vi "InitShooter.vi"   [LabVIEW 2020]
doc: "This VI initializes devices related directly to the shooter subsystem."
uses:
  <vilib>/Rock Robotics/WPI/ThirdParty/Phoenix-LabVIEW/Motor Controller/Controls/CTRE_Phoenix_MotorControl_NeutralMode.ctl
  <vilib>/Rock Robotics/WPI/ThirdParty/Phoenix-LabVIEW/Motor Controller/Controls/CTRE_Phoenix_MotorControl_TalonFXInvertType.ctl
  <vilib>/Rock Robotics/WPI/ThirdParty/Phoenix-LabVIEW/Motor Controller/Controls/CTRE_Phoenix_MotorControl_SupplyCurrentLimitConfiguration.ctl
  <vilib>/Rock Robotics/WPI/ThirdParty/Phoenix-LabVIEW/Motor Controller/Controls/CTRE_Phoenix_MotorControl_FeedbackDevice_TalonFX.ctl
  <vilib>/Rock Robotics/WPI/ThirdParty/Phoenix-LabVIEW/Motor Controller/Controls/CTRE_Phoenix_MotorControl_LimitSwitchSource_Local.ctl
  <vilib>/Rock Robotics/WPI/ThirdParty/Phoenix-LabVIEW/Motor Controller/Controls/CTRE_Phoenix_MotorControl_LimitSwitchNormal.ctl
  <vilib>/Rock Robotics/WPI/ThirdParty/Phoenix-LabVIEW/Motor Controller/Controls/CTRE_Phoenix_MotorControl_StatusFrameEnhanced.ctl
  refnumbers.vi
  robotconstants.vi
types:
  T1 = typedef "CTRE_Phoenix_MotorControl_StatusFrameEnhanced.ctl" = u16
  T2 = typedef "CTRE_Phoenix_MotorControl_LimitSwitchNormal.ctl" = enum16{"Normally Open", "Normally Closed", "Disabled"}
  T3 = typedef "CTRE_Phoenix_MotorControl_LimitSwitchSource_Local.ctl" = enum16{"Feedback Connector", "Remote Talon SRX", "Remote CANifier", "Deactivated"}
  T4 = typedef "CTRE_Phoenix_MotorControl_FeedbackDevice_TalonFX.ctl" = i8
  T5 = typedef "CTRE_Phoenix_MotorControl_SupplyCurrentLimitConfiguration.ctl" = cluster{"Enable?":bool, "Current Limit":dbl, "Threshold Current":dbl, "Threshold Time":dbl}
  T6 = typedef "CTRE_Phoenix_MotorControl_NeutralMode.ctl" = enum8{"EEPROMSetting", "Override to Coast", "Override to Brake"}
  T7 = typedef "CTRE_Phoenix_MotorControl_TalonFXInvertType.ctl" = enum16{"Counter-Clockwise", "Clockwise"}
  T8 = typedef "WPI_MotorControlDeviceRef.ctl" = cluster{"DeviceStatus":errorcluster, "Type":T9, "PWM":cluster{"PWM Channel":T10, "DeadBand":T11}, "CAN":cluster{"Device Number":u8, "SetOutput VI Ref":variant, "GetOutput VI Ref":variant, "Enable VI Ref":variant, "Disable VI Ref":variant, "Data":variant}, "Invert":bool, "DIO PWM":cluster{"PWM \"Enable\" Channel":T10, "DIOChannel":T12, "PWM Rate":dbl}}
  T9 = typedef "WPI_MotorControlType.ctl" = enum16{"PWM", "CAN", "DIO PWM"}
  T10 = typedef "FPGA_DIOPWMChannel.ctl" = enum8{"PWM 0", "PWM 1", "PWM 2", "PWM 3", "PWM 4", "PWM 5", "PWM 6", "PWM 7", "PWM 8", "PWM 9", "PWM MXP 0", "PWM MXP 1", "PWM MXP 2", "PWM MXP 3", "PWM MXP 4", "PWM MXP 5", "PWM MXP 6", "PWM MXP 7", "PWM MXP 8", "PWM MXP 9", "Invalid"}
  T11 = typedef "WPI_PWMDeadband.ctl" = cluster{"Name":string, "maxPositivePwm":i32, "minPositivePwm":i32, "centerPwm":i32, "maxNegativePwm":i32, "minNegativePwm":i32, "angularRange":u16}
  T12 = typedef "FPGA_DIOChannel.ctl" = enum8{"DIO 0", "DIO 1", "DIO 2", "DIO 3", "DIO 4", "DIO 5", "DIO 6", "DIO 7", "DIO 8", "DIO 9", "DIO MXP 0", "DIO MXP 1", "DIO MXP 2", "DIO MXP 3", "DIO MXP 4", "DIO MXP 5", "DIO MXP 6", "DIO MXP 7", "DIO MXP 8", "DIO MXP 9", "DIO MXP 10", "DIO MXP 11", "DIO MXP 12", "DIO MXP 13", "DIO MXP 14", "DIO MXP 15", "SPI Port CS1", "SPI Port CS2", "SPI Port CS3", "SPI Port MISO", "SPI Port MOSI", "Invalid"}
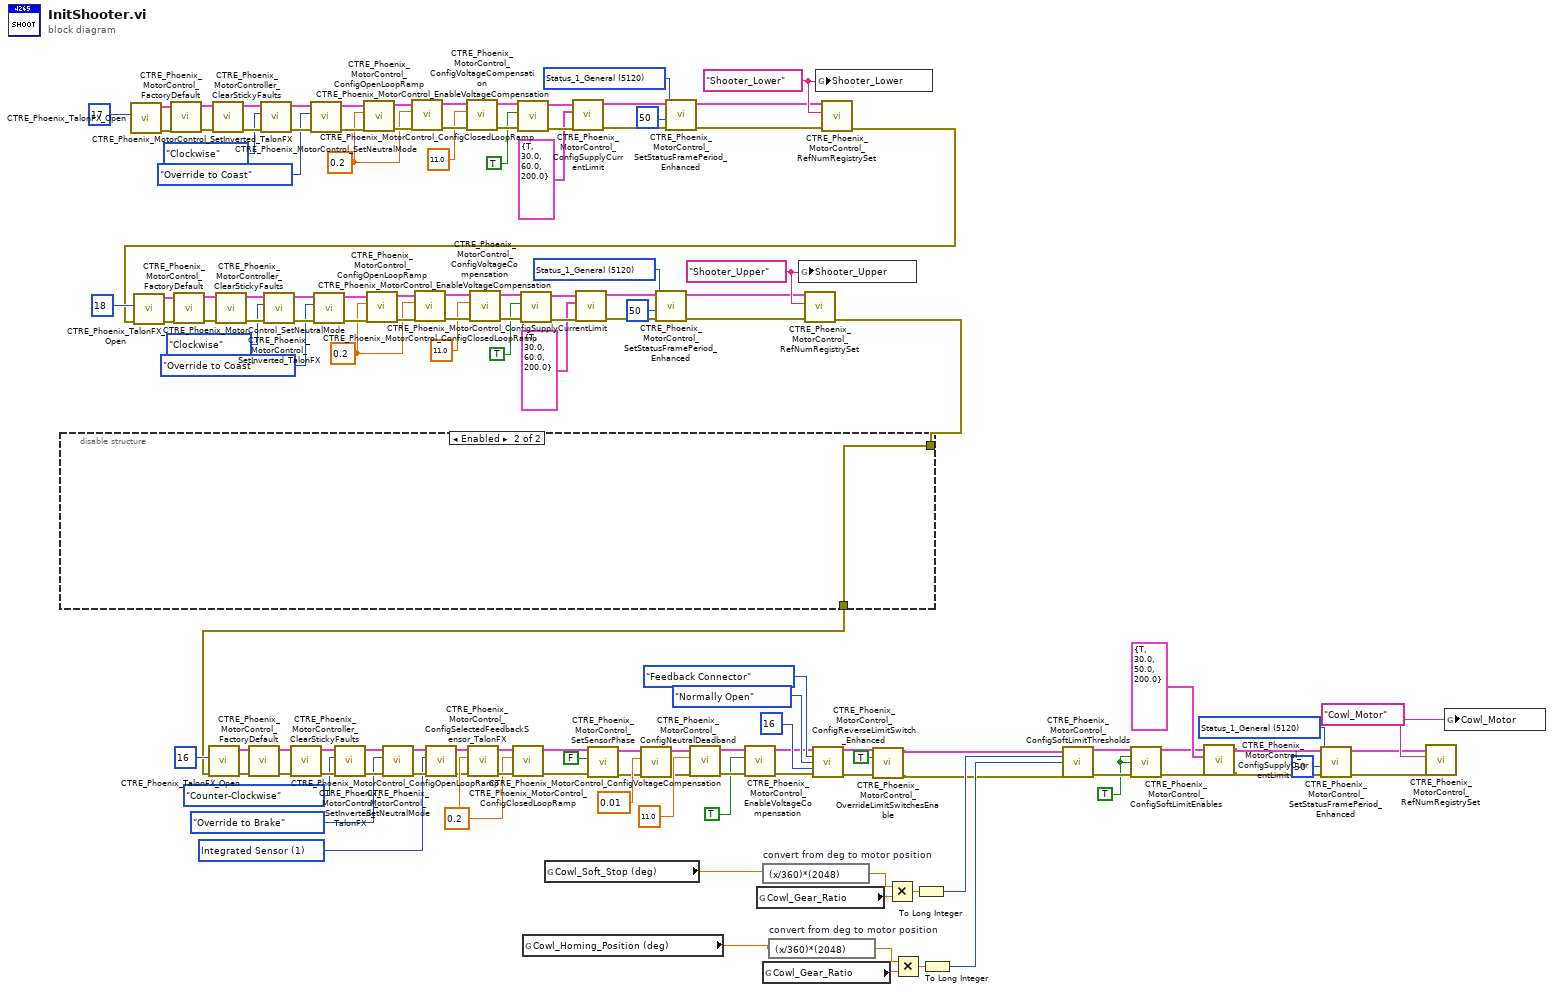
[diagram p0: block diagram]
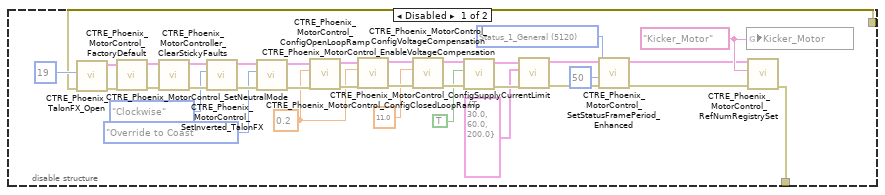
[diagram p2: hidden frame]
diagram:
  w17 = TRUE ("Forward Soft Limit Enable")
  w29 = T1 5120 items=["Status_1_General"=5120, "Status_2_Feedback0"=5184, "Status_3_Quadrature"=5248, "Status_4_AinTempVbat"=5312, "Status_6_Misc"=5440, "Status_7_CommStatus"=5504, "Status_8_PulseWidth"=5568, "Status_9_MotProfBuffer"=5632, "Status_10_MotionMagic"=5696, "Status_11_UartGadgeteer"=5760, "Status_12_Feedback1"=5824, "Status_13_Base_PIDF0"=5888, "Status_14_Turn_PIDF1"=5952, "Status_15_FirmwareApiStatus"=6016, "Status_Brushless_Current"=4672] ("Status Frame")
  w35 = T1 5120 items=["Status_1_General"=5120, "Status_2_Feedback0"=5184, "Status_3_Quadrature"=5248, "Status_4_AinTempVbat"=5312, "Status_6_Misc"=5440, "Status_7_CommStatus"=5504, "Status_8_PulseWidth"=5568, "Status_9_MotProfBuffer"=5632, "Status_10_MotionMagic"=5696, "Status_11_UartGadgeteer"=5760, "Status_12_Feedback1"=5824, "Status_13_Base_PIDF0"=5888, "Status_14_Turn_PIDF1"=5952, "Status_15_FirmwareApiStatus"=6016, "Status_Brushless_Current"=4672] ("Status Frame")
  w41 = T1 5120 items=["Status_1_General"=5120, "Status_2_Feedback0"=5184, "Status_3_Quadrature"=5248, "Status_4_AinTempVbat"=5312, "Status_6_Misc"=5440, "Status_7_CommStatus"=5504, "Status_8_PulseWidth"=5568, "Status_9_MotProfBuffer"=5632, "Status_10_MotionMagic"=5696, "Status_11_UartGadgeteer"=5760, "Status_12_Feedback1"=5824, "Status_13_Base_PIDF0"=5888, "Status_14_Turn_PIDF1"=5952, "Status_15_FirmwareApiStatus"=6016, "Status_Brushless_Current"=4672] ("Status Frame")
  w56 = T4 1 items=["Integrated Sensor"=1, "Sensor Sum (S0 + S1)"=9, "Sensor Difference (D0 - D1)"=10, "Remote Source 0"=11, "Remote Source 1"=12, "None"=14, "Software Emulated"=15] ("Talon FX Feedback Device")
  w62 = 0.2 ("secondsFromNeutralToFull")
  w76 = "Cowl_Motor" ("refnum name")
  w80 = "Shooter_Upper" ("refnum name")
  w90 = 0.2 ("secondsFromNeutralToFull")
  w106 = "Shooter_Lower" ("refnum name")
  w116 = 0.2 ("secondsFromNeutralToFull")
  n1 = call <vilib>:"CTRE_Phoenix_TalonFX_Open.vi"("Device Number"=u8 17) -> ("error out"=w130:errorcluster, "PhoenixMotorControlDevRef"=w129:T8)  [unwired: 9 in]
  n2 = call <vilib>:"CTRE_Phoenix_MotorControl_FactoryDefault.vi"("error in"=w130, "PhoenixMotorControlDevRef"=w129) -> ("error out"=w128:errorcluster, "PhoenixMotorControlDevRef"=w127:T8)  [unwired: 8 in]
  n3 = call <vilib>:"CTRE_Phoenix_MotorController_ClearStickyFaults.vi"("error in"=w128, "PhoenixMotorControlDevRef"=w127) -> ("error out"=w126:errorcluster, "PhoenixMotorControlDevRef"=w125:T8)  [unwired: 8 in]
  n4 = call <vilib>:"CTRE_Phoenix_MotorControl_SetInverted_TalonFX.vi"("error in (no error)"=w126, "Invert Type"=CTRE_Phoenix_MotorControl_TalonFXInvertType."Clockwise", "PhoenixMotorControlDevRef"=w125) -> ("error out"=w123:errorcluster, "PhoenixMotorControlDevRef"=w122:T8)  [unwired: 7 in]
  n5 = call <vilib>:"CTRE_Phoenix_MotorControl_SetNeutralMode.vi"("error in (no error)"=w123, "Motor Control Neutral Mode"=CTRE_Phoenix_MotorControl_NeutralMode."Override to Coast", "PhoenixMotorControlDevRef"=w122) -> ("error out"=w120:errorcluster, "PhoenixMotorControlDevRef"=w119:T8)  [unwired: 7 in]
  n6 = call <vilib>:"CTRE_Phoenix_MotorControl_ConfigOpenLoopRamp.vi"("error in (no error)"=w120, "secondsFromNeutralToFull"=w116, "PhoenixMotorControlDevRef"=w119) -> ("error out"=w118:errorcluster, "PhoenixMotorControlDevRef"=w117:T8)  [unwired: 7 in]
  n7 = call <vilib>:"CTRE_Phoenix_MotorControl_ConfigClosedLoopRamp.vi"("error in (no error)"=w118, "secondsFromNeutralToFull"=w116, "PhoenixMotorControlDevRef"=w117) -> ("error out"=w115:errorcluster, "PhoenixMotorControlDevRef"=w114:T8)  [unwired: 7 in]
  n8 = call <vilib>:"CTRE_Phoenix_MotorControl_ConfigVoltageCompensation.vi"("error in (no error)"=w115, "Saturation Voltage"=11.0, "PhoenixMotorControlDevRef"=w114) -> ("error out"=w112:errorcluster, "PhoenixMotorControlDevRef"=w111:T8)  [unwired: 7 in]
  n9 = call <vilib>:"CTRE_Phoenix_MotorControl_EnableVoltageCompensation.vi"("error in (no error)"=w112, "Enable Voltage Compensation?"=TRUE, "PhoenixMotorControlDevRef"=w111) -> ("error out"=w109:errorcluster, "PhoenixMotorControlDevRef"=w108:T8)  [unwired: 7 in]
  n10 = global read "robotconstants.vi" "Cowl_Homing_Position (deg)"() -> (w4:dbl)
  n11 = global read "robotconstants.vi" "Cowl_Soft_Stop (deg)"() -> (w3:dbl)
  n12 = call <vilib>:"CTRE_Phoenix_MotorControl_ConfigSupplyCurrentLimit.vi"("error in (no error)"=w109, "Supply Current Limit Configuration"=T5 {"Enable?"=TRUE, "Current Limit"=30.0, "Threshold Current"=60.0, "Threshold Time"=200.0}, "PhoenixMotorControlDevRef"=w108) -> ("error out"=w39:errorcluster, "PhoenixMotorControlDevRef"=w40:T8)  [unwired: 7 in]
  n13 = call <vilib>:"CTRE_Phoenix_MotorControl_SetStatusFramePeriod_Enhanced.vi"("error in (no error)"=w39, "periodMs"=50, "Status Frame"=w41, "PhoenixMotorControlDevRef"=w40) -> ("error out"=w37:errorcluster, "PhoenixMotorControlDevRef"=w38:T8)  [unwired: 6 in]
  n14 = global read "robotconstants.vi" "Cowl_Gear_Ratio"() -> (w14:dbl)
  n15 = expression code="(x/360)*(2048)" "convert from deg to motor position"(w3) -> (w16:dbl)
  n16 = global read "robotconstants.vi" "Cowl_Gear_Ratio"() -> (w11:dbl)
  n17 = expression code="(x/360)*(2048)" "convert from deg to motor position"(w4) -> (w13:dbl)
  n18 = global write "refnumbers.vi" "Shooter_Upper"(w80) -> ()
  n19 = global write "refnumbers.vi" "Shooter_Lower"(w106) -> ()
  n20 = call <vilib>:"CTRE_Phoenix_MotorControl_RefNumRegistrySet.vi"("error in (no error)"=w37, "refnum name"=w106, "PhoenixMotorControlDevRef"=w38) -> ("error out"=w79:errorcluster)  [unwired: 7 in, 1 out]
  n21 = call <vilib>:"CTRE_Phoenix_TalonFX_Open.vi"("error in"=w79, "Device Number"=u8 18) -> ("error out"=w104:errorcluster, "PhoenixMotorControlDevRef"=w103:T8)  [unwired: 8 in]
  n22 = call <vilib>:"CTRE_Phoenix_MotorControl_FactoryDefault.vi"("error in"=w104, "PhoenixMotorControlDevRef"=w103) -> ("error out"=w102:errorcluster, "PhoenixMotorControlDevRef"=w101:T8)  [unwired: 8 in]
  n23 = call <vilib>:"CTRE_Phoenix_MotorController_ClearStickyFaults.vi"("error in"=w102, "PhoenixMotorControlDevRef"=w101) -> ("error out"=w100:errorcluster, "PhoenixMotorControlDevRef"=w99:T8)  [unwired: 8 in]
  n24 = call <vilib>:"CTRE_Phoenix_MotorControl_SetInverted_TalonFX.vi"("error in (no error)"=w100, "Invert Type"=CTRE_Phoenix_MotorControl_TalonFXInvertType."Clockwise", "PhoenixMotorControlDevRef"=w99) -> ("error out"=w97:errorcluster, "PhoenixMotorControlDevRef"=w96:T8)  [unwired: 7 in]
  n25 = call <vilib>:"CTRE_Phoenix_MotorControl_SetNeutralMode.vi"("error in (no error)"=w97, "Motor Control Neutral Mode"=CTRE_Phoenix_MotorControl_NeutralMode."Override to Coast", "PhoenixMotorControlDevRef"=w96) -> ("error out"=w94:errorcluster, "PhoenixMotorControlDevRef"=w93:T8)  [unwired: 7 in]
  n26 = call <vilib>:"CTRE_Phoenix_MotorControl_ConfigOpenLoopRamp.vi"("error in (no error)"=w94, "secondsFromNeutralToFull"=w90, "PhoenixMotorControlDevRef"=w93) -> ("error out"=w92:errorcluster, "PhoenixMotorControlDevRef"=w91:T8)  [unwired: 7 in]
  n27 = call <vilib>:"CTRE_Phoenix_MotorControl_ConfigClosedLoopRamp.vi"("error in (no error)"=w92, "secondsFromNeutralToFull"=w90, "PhoenixMotorControlDevRef"=w91) -> ("error out"=w89:errorcluster, "PhoenixMotorControlDevRef"=w88:T8)  [unwired: 7 in]
  n28 = call <vilib>:"CTRE_Phoenix_MotorControl_ConfigVoltageCompensation.vi"("error in (no error)"=w89, "Saturation Voltage"=11.0, "PhoenixMotorControlDevRef"=w88) -> ("error out"=w86:errorcluster, "PhoenixMotorControlDevRef"=w85:T8)  [unwired: 7 in]
  n29 = call <vilib>:"CTRE_Phoenix_MotorControl_EnableVoltageCompensation.vi"("error in (no error)"=w86, "Enable Voltage Compensation?"=TRUE, "PhoenixMotorControlDevRef"=w85) -> ("error out"=w83:errorcluster, "PhoenixMotorControlDevRef"=w82:T8)  [unwired: 7 in]
  n30 = call <vilib>:"CTRE_Phoenix_MotorControl_ConfigSupplyCurrentLimit.vi"("error in (no error)"=w83, "Supply Current Limit Configuration"=T5 {"Enable?"=TRUE, "Current Limit"=30.0, "Threshold Current"=60.0, "Threshold Time"=200.0}, "PhoenixMotorControlDevRef"=w82) -> ("error out"=w33:errorcluster, "PhoenixMotorControlDevRef"=w34:T8)  [unwired: 7 in]
  n31 = call <vilib>:"CTRE_Phoenix_MotorControl_SetStatusFramePeriod_Enhanced.vi"("error in (no error)"=w33, "periodMs"=50, "Status Frame"=w35, "PhoenixMotorControlDevRef"=w34) -> ("error out"=w31:errorcluster, "PhoenixMotorControlDevRef"=w32:T8)  [unwired: 6 in]
  n32 = call <vilib>:"CTRE_Phoenix_MotorControl_RefNumRegistrySet.vi"("error in (no error)"=w31, "refnum name"=w80, "PhoenixMotorControlDevRef"=w32) -> ("error out"=w2:errorcluster)  [unwired: 7 in, 1 out]
  n33 = disable-structure shown="Enabled" {
    disable-tunnel: w2 -> [w133 w166]
    disable-tunnel: [w132 w166] -> w1
    frame Disabled {
      w138 = T1 5120 items=["Status_1_General"=5120, "Status_2_Feedback0"=5184, "Status_3_Quadrature"=5248, "Status_4_AinTempVbat"=5312, "Status_6_Misc"=5440, "Status_7_CommStatus"=5504, "Status_8_PulseWidth"=5568, "Status_9_MotProfBuffer"=5632, "Status_10_MotionMagic"=5696, "Status_11_UartGadgeteer"=5760, "Status_12_Feedback1"=5824, "Status_13_Base_PIDF0"=5888, "Status_14_Turn_PIDF1"=5952, "Status_15_FirmwareApiStatus"=6016, "Status_Brushless_Current"=4672] ("Status Frame")
      w140 = "Kicker_Motor" ("refnum name")
      w150 = 0.2 ("secondsFromNeutralToFull")
      n34 = call <vilib>:"CTRE_Phoenix_TalonFX_Open.vi"("error in"=w133, "Device Number"=u8 19) -> ("error out"=w164:errorcluster, "PhoenixMotorControlDevRef"=w163:T8)  [unwired: 8 in]
      n35 = call <vilib>:"CTRE_Phoenix_MotorControl_FactoryDefault.vi"("error in"=w164, "PhoenixMotorControlDevRef"=w163) -> ("error out"=w162:errorcluster, "PhoenixMotorControlDevRef"=w161:T8)  [unwired: 8 in]
      n36 = call <vilib>:"CTRE_Phoenix_MotorController_ClearStickyFaults.vi"("error in"=w162, "PhoenixMotorControlDevRef"=w161) -> ("error out"=w160:errorcluster, "PhoenixMotorControlDevRef"=w159:T8)  [unwired: 8 in]
      n37 = call <vilib>:"CTRE_Phoenix_MotorControl_SetInverted_TalonFX.vi"("error in (no error)"=w160, "Invert Type"=CTRE_Phoenix_MotorControl_TalonFXInvertType."Clockwise", "PhoenixMotorControlDevRef"=w159) -> ("error out"=w157:errorcluster, "PhoenixMotorControlDevRef"=w156:T8)  [unwired: 7 in]
      n38 = call <vilib>:"CTRE_Phoenix_MotorControl_SetNeutralMode.vi"("error in (no error)"=w157, "Motor Control Neutral Mode"=CTRE_Phoenix_MotorControl_NeutralMode."Override to Coast", "PhoenixMotorControlDevRef"=w156) -> ("error out"=w154:errorcluster, "PhoenixMotorControlDevRef"=w153:T8)  [unwired: 7 in]
      n39 = call <vilib>:"CTRE_Phoenix_MotorControl_ConfigOpenLoopRamp.vi"("error in (no error)"=w154, "secondsFromNeutralToFull"=w150, "PhoenixMotorControlDevRef"=w153) -> ("error out"=w152:errorcluster, "PhoenixMotorControlDevRef"=w151:T8)  [unwired: 7 in]
      n40 = call <vilib>:"CTRE_Phoenix_MotorControl_ConfigClosedLoopRamp.vi"("error in (no error)"=w152, "secondsFromNeutralToFull"=w150, "PhoenixMotorControlDevRef"=w151) -> ("error out"=w149:errorcluster, "PhoenixMotorControlDevRef"=w148:T8)  [unwired: 7 in]
      n41 = call <vilib>:"CTRE_Phoenix_MotorControl_ConfigVoltageCompensation.vi"("error in (no error)"=w149, "Saturation Voltage"=11.0, "PhoenixMotorControlDevRef"=w148) -> ("error out"=w146:errorcluster, "PhoenixMotorControlDevRef"=w145:T8)  [unwired: 7 in]
      n42 = call <vilib>:"CTRE_Phoenix_MotorControl_EnableVoltageCompensation.vi"("error in (no error)"=w146, "Enable Voltage Compensation?"=TRUE, "PhoenixMotorControlDevRef"=w145) -> ("error out"=w143:errorcluster, "PhoenixMotorControlDevRef"=w142:T8)  [unwired: 7 in]
      n43 = call <vilib>:"CTRE_Phoenix_MotorControl_ConfigSupplyCurrentLimit.vi"("error in (no error)"=w143, "Supply Current Limit Configuration"=T5 {"Enable?"=TRUE, "Current Limit"=30.0, "Threshold Current"=60.0, "Threshold Time"=200.0}, "PhoenixMotorControlDevRef"=w142) -> ("error out"=w136:errorcluster, "PhoenixMotorControlDevRef"=w137:T8)  [unwired: 7 in]
      n44 = call <vilib>:"CTRE_Phoenix_MotorControl_SetStatusFramePeriod_Enhanced.vi"("error in (no error)"=w136, "periodMs"=50, "Status Frame"=w138, "PhoenixMotorControlDevRef"=w137) -> ("error out"=w134:errorcluster, "PhoenixMotorControlDevRef"=w135:T8)  [unwired: 6 in]
      n45 = global write "refnumbers.vi" "Kicker_Motor"(w140) -> ()
      n46 = call <vilib>:"CTRE_Phoenix_MotorControl_RefNumRegistrySet.vi"("error in (no error)"=w134, "refnum name"=w140, "PhoenixMotorControlDevRef"=w135) -> ("error out"=w132:errorcluster)  [unwired: 7 in, 1 out]
    }
    frame Enabled {
    }
  }
  n47 = call <vilib>:"CTRE_Phoenix_TalonFX_Open.vi"("error in"=w1, "Device Number"=u8 16 ("Drive 4L")) -> ("error out"=w67:errorcluster, "PhoenixMotorControlDevRef"=w74:T8)  [unwired: 8 in]
  n48 = call <vilib>:"CTRE_Phoenix_MotorControl_FactoryDefault.vi"("error in"=w67, "PhoenixMotorControlDevRef"=w74) -> ("error out"=w70:errorcluster, "PhoenixMotorControlDevRef"=w71:T8)  [unwired: 8 in]
  n49 = call <vilib>:"CTRE_Phoenix_MotorController_ClearStickyFaults.vi"("error in"=w70, "PhoenixMotorControlDevRef"=w71) -> ("error out"=w69:errorcluster, "PhoenixMotorControlDevRef"=w68:T8)  [unwired: 8 in]
  n50 = call <vilib>:"CTRE_Phoenix_MotorControl_SetInverted_TalonFX.vi"("error in (no error)"=w69, "Invert Type"=CTRE_Phoenix_MotorControl_TalonFXInvertType."Counter-Clockwise", "PhoenixMotorControlDevRef"=w68) -> ("error out"=w77:errorcluster, "PhoenixMotorControlDevRef"=w78:T8)  [unwired: 7 in]
  n51 = call <vilib>:"CTRE_Phoenix_MotorControl_SetNeutralMode.vi"("error in (no error)"=w77, "Motor Control Neutral Mode"=CTRE_Phoenix_MotorControl_NeutralMode."Override to Brake", "PhoenixMotorControlDevRef"=w78) -> ("error out"=w65:errorcluster, "PhoenixMotorControlDevRef"=w66:T8)  [unwired: 7 in]
  n52 = call <vilib>:"CTRE_Phoenix_MotorControl_ConfigSelectedFeedbackSensor_TalonFX.vi"("error in (no error)"=w65, "Talon FX Feedback Device"=w56, "PhoenixMotorControlDevRef"=w66) -> ("error out"=w50:errorcluster, "PhoenixMotorControlDevRef"=w51:T8)  [unwired: 7 in]
  n53 = call <vilib>:"CTRE_Phoenix_MotorControl_ConfigOpenLoopRamp.vi"("error in (no error)"=w50, "secondsFromNeutralToFull"=w62, "PhoenixMotorControlDevRef"=w51) -> ("error out"=w72:errorcluster, "PhoenixMotorControlDevRef"=w73:T8)  [unwired: 7 in]
  n54 = call <vilib>:"CTRE_Phoenix_MotorControl_ConfigClosedLoopRamp.vi"("error in (no error)"=w72, "secondsFromNeutralToFull"=w62, "PhoenixMotorControlDevRef"=w73) -> ("error out"=w48:errorcluster, "PhoenixMotorControlDevRef"=w49:T8)  [unwired: 7 in]
  n55 = call <vilib>:"CTRE_Phoenix_MotorControl_SetSensorPhase.vi"("error in (no error)"=w48, "PhaseSensor"=FALSE, "PhoenixMotorControlDevRef"=w49) -> ("error out"=w22:errorcluster, "PhoenixMotorControlDevRef"=w23:T8)  [unwired: 7 in]
  n56 = call <vilib>:"CTRE_Phoenix_MotorControl_ConfigNeutralDeadband.vi"("error in (no error)"=w22, "Percent Deadband"=0.01, "PhoenixMotorControlDevRef"=w23) -> ("error out"=w20:errorcluster, "PhoenixMotorControlDevRef"=w21:T8)  [unwired: 7 in]
  n57 = call <vilib>:"CTRE_Phoenix_MotorControl_ConfigVoltageCompensation.vi"("error in (no error)"=w20, "Saturation Voltage"=11.0, "PhoenixMotorControlDevRef"=w21) -> ("error out"=w60:errorcluster, "PhoenixMotorControlDevRef"=w61:T8)  [unwired: 7 in]
  n58 = call <vilib>:"CTRE_Phoenix_MotorControl_EnableVoltageCompensation.vi"("error in (no error)"=w60, "Enable Voltage Compensation?"=TRUE, "PhoenixMotorControlDevRef"=w61) -> ("error out"=w45:errorcluster, "PhoenixMotorControlDevRef"=w46:T8)  [unwired: 7 in]
  n59 = call <vilib>:"CTRE_Phoenix_MotorControl_ConfigReverseLimitSwitch_Enhanced.vi"("PhoenixMotorControlDevRef"=w46, "Limit Switch Source"=CTRE_Phoenix_MotorControl_LimitSwitchSource_Local."Feedback Connector", "NormallyOpenOrClosed"=CTRE_Phoenix_MotorControl_LimitSwitchNormal."Normally Open", "deviceID"=16, "error in (no error)"=w45) -> ("PhoenixMotorControlDevRef"=w44:T8, "error out"=w43:errorcluster)  [unwired: 9 in]
  n60 = call <vilib>:"CTRE_Phoenix_MotorControl_OverrideLimitSwitchesEnable.vi"("PhoenixMotorControlDevRef"=w44, "Override Limit Switch Enable?"=TRUE, "error in (no error)"=w43) -> ("PhoenixMotorControlDevRef"=w8:T8, "error out"=w7:errorcluster)  [unwired: 11 in]
  n61 = Multiply(x=w16, y=w14) -> (x*y=w15:dbl)
  n62 = Multiply(x=w13, y=w11) -> (x*y=w12:dbl)
  n63 = To Long Integer(number=w15) -> (32bit integer=w10:i32)
  n64 = To Long Integer(number=w12) -> (32bit integer=w9:i32)
  n65 = call <vilib>:"CTRE_Phoenix_MotorControl_ConfigSoftLimitThresholds.vi"("PhoenixMotorControlDevRef"=w8, "Forward Soft Limit"=w10, "Reverse Soft Limit"=w9, "error in (no error)"=w7) -> ("PhoenixMotorControlDevRef"=w18:T8, "error out"=w19:errorcluster)  [unwired: 10 in]
  n66 = call <vilib>:"CTRE_Phoenix_MotorControl_ConfigSoftLimitEnables.vi"("PhoenixMotorControlDevRef"=w18, "Forward Soft Limit Enable"=w17, "Reverse Soft Limit Enable"=w17, "error in (no error)"=w19) -> ("PhoenixMotorControlDevRef"=w6:T8, "error out"=w5:errorcluster)  [unwired: 10 in]
  n67 = call <vilib>:"CTRE_Phoenix_MotorControl_ConfigSupplyCurrentLimit.vi"("error in (no error)"=w5, "Supply Current Limit Configuration"=T5 {"Enable?"=TRUE, "Current Limit"=30.0, "Threshold Current"=50.0, "Threshold Time"=200.0}, "PhoenixMotorControlDevRef"=w6) -> ("error out"=w27:errorcluster, "PhoenixMotorControlDevRef"=w28:T8)  [unwired: 7 in]
  n68 = call <vilib>:"CTRE_Phoenix_MotorControl_SetStatusFramePeriod_Enhanced.vi"("error in (no error)"=w27, "periodMs"=50, "Status Frame"=w29, "PhoenixMotorControlDevRef"=w28) -> ("error out"=w25:errorcluster, "PhoenixMotorControlDevRef"=w26:T8)  [unwired: 6 in]
  n69 = call <vilib>:"CTRE_Phoenix_MotorControl_RefNumRegistrySet.vi"("error in (no error)"=w25, "refnum name"=w76, "PhoenixMotorControlDevRef"=w26) -> ()  [unwired: 7 in, 2 out]
  n70 = global write "refnumbers.vi" "Cowl_Motor"(w76) -> ()
